vi "Test Counter.vi"(4 "#C":i32, 6 "C Counter":i32, 8 "#B":i32, 9 "B Counter":i32, 10 "#A":i32, 11 "A Counter in":i32) -> (0 "Next (T)":bool, 1 "C Counter out":i32, 2 "B Counter out":i32, 3 "A Counter out":i32)   [LabVIEW 2017]
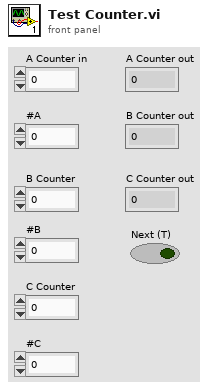
[diagram p1: front panel]
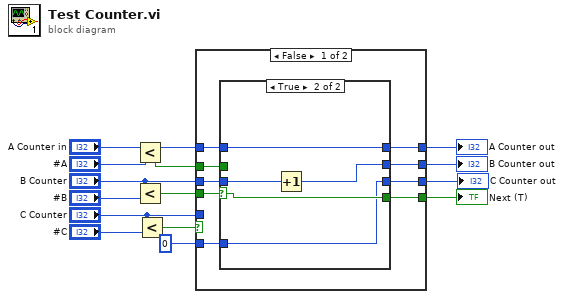
[diagram p0: block diagram]
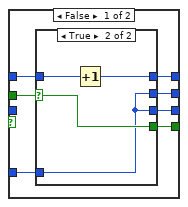
[diagram p2: hidden frame]
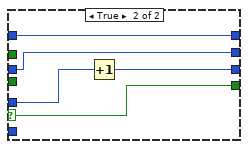
[diagram p4: hidden frame]
diagram:
  n1 = Less?(x="A Counter in", y="#A") -> (x < y?=w12:bool)
  n2 = Less?(x="B Counter", y="#B") -> (x < y?=w13:bool)
  n3 = Less?(x="C Counter", y="#C") -> (x < y?=w2:bool)
  n4 = case shown="False" w2 {
    selector: w2 -> [_ w42]
    tunnel: [w23 w42] -> w14
    tunnel: w13 -> [w22 _]
    tunnel: w12 -> [w21 _]
    tunnel: [w20 w44] -> w11
    tunnel: [w19 w43] -> w10
    tunnel: "B Counter" -> [w18 w44]
    tunnel: 0 -> [w17 _]
    tunnel: "A Counter in" -> [w16 w43]
    tunnel: "C Counter" -> [_ w46]
    tunnel: [w15 w45] -> w1
    frame False {
      n5 = case shown="True" w22 {
        selector: w22 -> [_ w38]
        tunnel: w16 -> [w29 w41]
        tunnel: w21 -> [w30 _]
        tunnel: [w28 w41] -> w19
        tunnel: [w27 w39] -> w20
        tunnel: w17 -> [w26 w37]
        tunnel: w18 -> [_ w40]
        tunnel: [w25 w38] -> w23
        tunnel: [w24 w37] -> w15
        frame False {
          n6 = case shown="True" w30 {
            selector: w30 -> [w32 w34]
            tunnel: w29 -> [_ w36]
            tunnel: [w31 w35] -> w28
            tunnel: [w31 w33] -> w27
            tunnel: w26 -> [w31 w33]
            tunnel: [w32 w34] -> w25
            tunnel: [w31 w33] -> w24
            frame False {
            }
            frame True {
              n7 = Increment(x=w36) -> (x+1=w35:i32)
            }
          }
        }
        frame True {
          n8 = Increment(x=w40) -> (x+1=w39:i32)
        }
      }
    }
    frame True {
      n9 = Increment(x=w46) -> (x+1=w45:i32)
    }
  }
  "Next (T)" <- w14
  "B Counter out" <- w11
  "A Counter out" <- w10
  "C Counter out" <- w1
